vi "CODMn插入数据.vi"(1 "data":T3 {"单位" items=["ug/L", "mg/L", "ppm", "mg/m3", "cm", "ppb", "ug/m3", "%", "nmol/mol", "umol/mol", "MPN/L", "MPN/100ml", "ng/m3", "NTU", "无量纲", "ms/cm", "us/cm"]}, 2 "CODMn关键参数":T2, 3 "SN":string, 5 "table":string, 7 "测量模式":T4(ring)=enum."水样测试", 9 "数据类型":string(combo)="N", 11 "error in (no error)":errorcluster) -> (15 "error out":errorcluster)   [LabVIEW 2016, in "斯坦道CODMn新电路板.lvlib"]
uses:
  <vilib>/Utility/error.llb/DialogType.ctl
panel:
  in  "data 2":T1={"时间"=timestamp(0 s since 1904-01-01), "测量模式"="水样测试", "数据类型"="N", "检测值"=0.0, "单位"="mg/L", "数据标识"="N", "终点滴定数"=0.0, "量程"=0.0, "SN"="", "标样参考值"=0.0, "跨度值"=0.0, "A"=0, "B"=0, "K"=0, "环境温度"=0.0, "加热实时温度"=0.0, "因子编码"="", "X0"=0.0, "X^2"=0.0, "X"=0.0, "B 2"=0.0, "光值1"=0.0, "光值2"=0.0, "光值3"=0.0, "光值4"=0.0, "光值5"=0.0, "光值6"=0.0, "光值7"=0.0, "光值8"=0.0, "测量量程"=0.0, "测量检出限"=0.0, "测量精度"=0.0, "测量间隔"=0.0, "消解温度"=0.0, "消解时长"=0.0, "三项式系数"=0.0, "二次多项式系数"=0.0, "曲线斜率"=0.0, "曲线截距"=0.0, "线性相关系数"=0.0, "空白校准时间"=timestamp(0 s since 1904-01-01), "标样校准时间"=timestamp(0 s since 1904-01-01), "测量信号值"=0.0, "稀释倍数"=0.0, "量程系数"=0.0, "LastTime"=timestamp(0 s since 1904-01-01)}
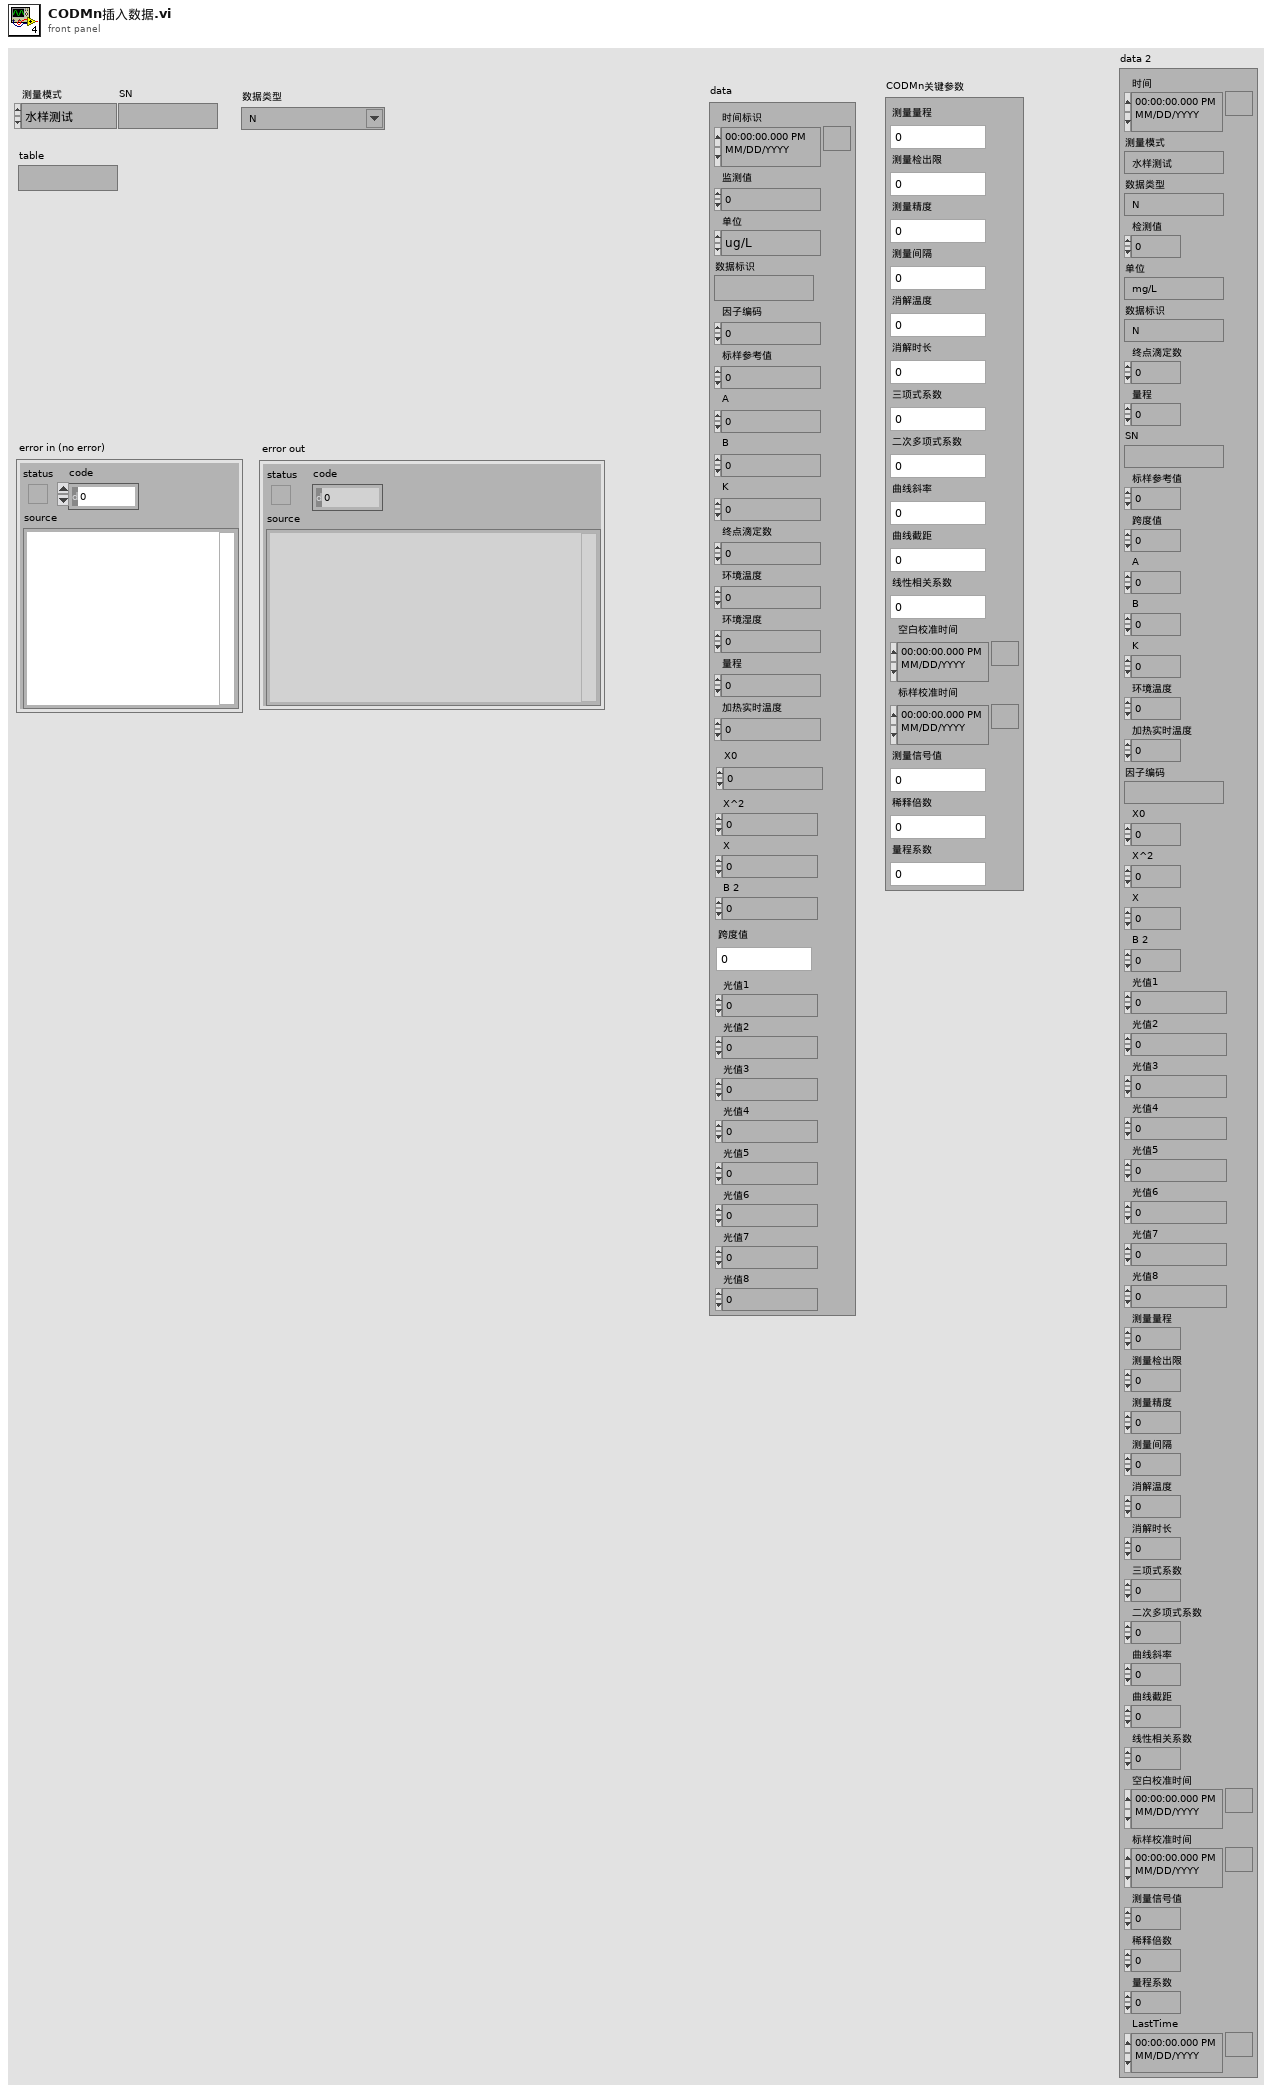
[diagram p1: front panel]
types:
  T1 = cluster{"时间":timestamp, "测量模式":string, "数据类型":string, "检测值":sgl, "单位":string, "数据标识":string, "终点滴定数":sgl, "量程":sgl, "SN":string, "标样参考值":sgl, "跨度值":sgl, "A":u32, "B":u32, "K":u32, "环境温度":sgl, "加热实时温度":sgl, "因子编码":string, "X0":sgl, "X^2":sgl, "X":sgl, "B 2":sgl, "光值1":sgl, "光值2":sgl, "光值3":sgl, "光值4":sgl, "光值5":sgl, "光值6":sgl, "光值7":sgl, "光值8":sgl, "测量量程":sgl, "测量检出限":sgl, "测量精度":sgl, "测量间隔":sgl, "消解温度":sgl, "消解时长":sgl, "三项式系数":sgl, "二次多项式系数":sgl, "曲线斜率":sgl, "曲线截距":sgl, "线性相关系数":sgl, "空白校准时间":timestamp, "标样校准时间":timestamp, "测量信号值":sgl, "稀释倍数":sgl, "量程系数":sgl, "LastTime":timestamp}
  T2 = cluster{"测量量程":sgl, "测量检出限":sgl, "测量精度":sgl, "测量间隔":sgl, "消解温度":sgl, "消解时长":sgl, "三项式系数":sgl, "二次多项式系数":sgl, "曲线斜率":sgl, "曲线截距":sgl, "线性相关系数":sgl, "空白校准时间":timestamp, "标样校准时间":timestamp, "测量信号值":sgl, "稀释倍数":sgl, "量程系数":sgl}
  T3 = cluster{"时间标识":timestamp, "监测值":sgl, "单位":u16, "数据标识":string, "因子编码":u32, "标样参考值":sgl, "A":sgl, "B":sgl, "K":sgl, "终点滴定数":sgl, "环境温度":sgl, "环境湿度":sgl, "量程":sgl, "加热实时温度":sgl, "X0":sgl, "X^2":sgl, "X":sgl, "B 2":sgl, "跨度值":sgl, "光值1":sgl, "光值2":sgl, "光值3":sgl, "光值4":sgl, "光值5":sgl, "光值6":sgl, "光值7":sgl, "光值8":sgl}
  T4 = enum16{"维护数据", "水样测试", "标样核查", "零点核查", "跨度核查", "空白测试", "平行样测试", "加标回收", "空白校准", "标样校准", "初始化（清洗）"}
  T5 = typedef "DialogType.ctl" = u16
  T6 = typedef "数据库类型.ctl" = enum16{"Access", "SQLite"}
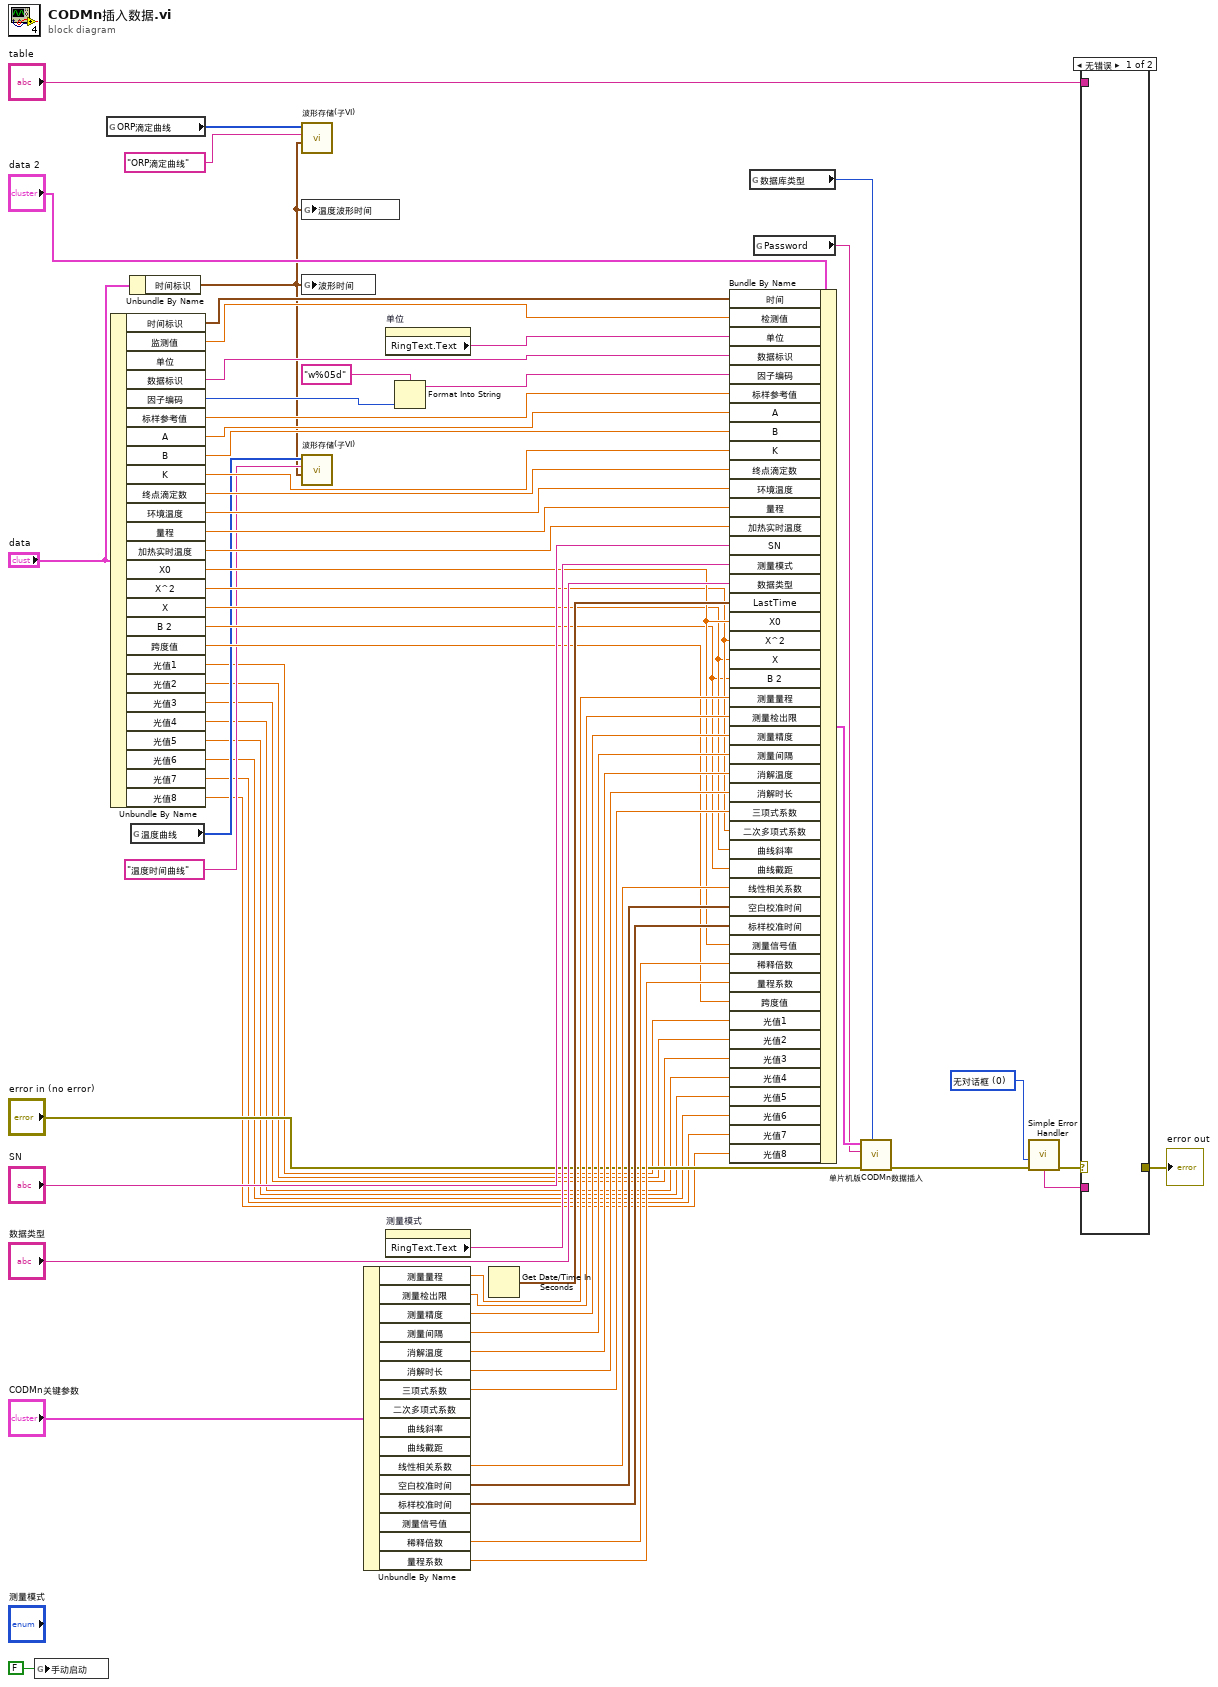
[diagram p0: block diagram]
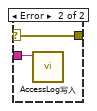
[diagram p2: hidden frame]
diagram:
  w63 = T5 0 items=["无对话框", "确定信息", "继续或停止信息", "确定信息＋警告", "继续/停止+警告"] ("type of dialog (OK msg:1)")
  n1 = global write "VARCODMn全局变量.vi" "手动启动"(FALSE ("手动启动")) -> ()
  n2 = global read "VARCODMn全局变量.vi" "ORP滴定曲线"() -> (w18:u16[])
  n3 = Unbundle By Name("data") -> ("时间标识"=w39:timestamp, "监测值"=w57:sgl, "数据标识"=w55:string, "因子编码"=w53:u32, "标样参考值"=w51:sgl, "A"=w50:sgl, "B"=w49:sgl, "K"=w48:sgl, "终点滴定数"=w47:sgl, "环境温度"=w46:sgl, "量程"=w45:sgl, "加热实时温度"=w44:sgl, "X0"=w28:sgl, "X^2"=w23:sgl, "X"=w22:sgl, "B 2"=w21:sgl, "跨度值"=w24:sgl, "光值1"=w8:sgl, "光值2"=w7:sgl, "光值3"=w6:sgl, "光值4"=w5:sgl, "光值5"=w4:sgl, "光值6"=w3:sgl, "光值7"=w2:sgl, "光值8"=w1:sgl)  [unwired: 1 out]
  n4 = Unbundle By Name("data") -> ("时间标识"=w14:timestamp)
  n5 = global read "VARCODMn全局变量.vi" "温度曲线"() -> (w16:u16[])
  n6 = call "波形存储(子VI).vi"("波形时间"=w14, "condition"="ORP滴定曲线", "ORP滴定曲线"=w18) -> ()  [unwired: 9 in]
  n7 = global write "VARCODMn全局变量.vi" "温度波形时间"(w14) -> ()
  n8 = global write "VARCODMn全局变量.vi" "波形时间"(w14) -> ()
  n9 = call "波形存储(子VI).vi"("波形时间"=w14, "condition"="温度时间曲线", "ORP滴定曲线"=w16) -> ()  [unwired: 9 in]
  n10 = Unbundle By Name("CODMn关键参数") -> ("测量量程"=w38:sgl, "测量检出限"=w37:sgl, "测量精度"=w36:sgl, "测量间隔"=w35:sgl, "消解温度"=w34:sgl, "消解时长"=w33:sgl, "三项式系数"=w32:sgl, "线性相关系数"=w31:sgl, "空白校准时间"=w30:timestamp, "标样校准时间"=w29:timestamp, "稀释倍数"=w27:sgl, "量程系数"=w26:sgl)  [unwired: 4 out]
  n11 = property on="单位" class="Ring (严格)"() -> ("RingText.Text"=w56:string)  [unwired: 2 in, 2 out]
  n12 = property on="测量模式" class="Enum (严格)"() -> ("RingText.Text"=w42:string)  [unwired: 2 in, 2 out]
  n13 = Format Into String(format string="w%05d" ("格式字符串"), w53) -> (resulting string=w52:string)  [unwired: 2 in, 1 out]
  n14 = Get Date/Time In Seconds() -> (seconds since 1Jan1904=w40:timestamp)
  n15 = Bundle By Name(cluster="data 2", "时间"=w39, "检测值"=w57, "单位"=w56, "数据标识"=w55, "因子编码"=w52, "标样参考值"=w51, "A"=w50, "B"=w49, "K"=w48, "终点滴定数"=w47, "环境温度"=w46, "量程"=w45, "加热实时温度"=w44, "SN"="SN", "测量模式"=w42, "数据类型"="数据类型", "LastTime"=w40, "X0"=w28, "X^2"=w23, "X"=w22, "B 2"=w21, "测量量程"=w38, "测量检出限"=w37, "测量精度"=w36, "测量间隔"=w35, "消解温度"=w34, "消解时长"=w33, "三项式系数"=w32, "二次多项式系数"=w23, "曲线斜率"=w22, "曲线截距"=w21, "线性相关系数"=w31, "空白校准时间"=w30, "标样校准时间"=w29, "测量信号值"=w28, "稀释倍数"=w27, "量程系数"=w26, "跨度值"=w24, "光值1"=w8, "光值2"=w7, "光值3"=w6, "光值4"=w5, "光值5"=w4, "光值6"=w3, "光值7"=w2, "光值8"=w1) -> (w19:T1)
  n16 = global read "CODMn断电保存全局变量.vi" "数据库类型"() -> (w10:T6)
  n17 = global read "CODMn断电保存全局变量.vi" "Password"() -> (w9:string)
  n18 = call "单片机版CODMn数据插入.vi"("data"=w19, "Password"=w9, "错误输入（无错误）"="error in (no error)", "数据库类型"=w10) -> ("错误输出"=w12:errorcluster)  [unwired: 6 in]
  n19 = call <vilib>:"Simple Error Handler.vi"("type of dialog (OK msg:1)"=w63, "error in (no error)"=w12) -> ("error out"=w62:errorcluster, "message"=w61:string)  [unwired: 3 in, 3 out]
  n20 = case shown="无错误" w62 {
    selector: w62 -> [_ w64]
    tunnel: w61 -> [_ w65]
    tunnel: [_ w64] -> w60
    tunnel: "table" -> [_ _]
    frame No Error {
    }
    frame Error {
      n21 = call "AccessLog写入.vi"("Log"=w65) -> ()  [unwired: 11 in]
    }
  }
  "error out" <- w60
